vi "ti2_setYPos.vi"(8 "error in (no error)":errorcluster, 10 "speed":i32=4, 11 "y Position (um)":dbl) -> (0 "error out":errorcluster)   [LabVIEW 2018, in "ti2lv.lvlib"]
uses:
  ti2lv.lvlib
  ti2wrap/x64/Release/ti2wrap.dll
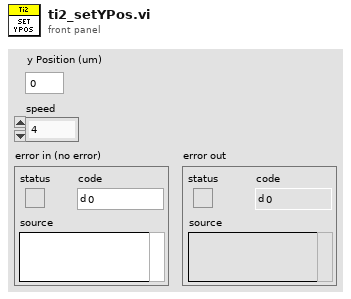
[diagram p1: front panel]
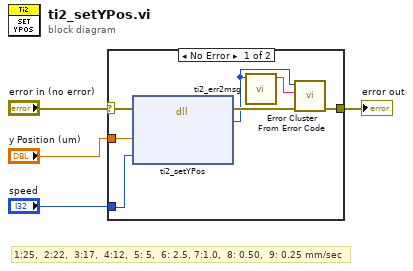
[diagram p0: block diagram]
diagram:
  # "1:25,  2:22, \t3:17,  4:12,\t\t5: 5,  6: 2.5,\t7:1.0,  8: 0.50,  9: 0.25 mm/sec"
  n1 = case shown="No Error" "error in (no error)" {
    selector: "error in (no error)" -> [w10 w12]
    tunnel: [w11 w12] -> w4
    tunnel: "y Position (um)" -> [w6 _]
    tunnel: "speed" -> [w5 _]
    frame No Error {
      n2 = dll-call lib="C:/LVCUR/Flash Gordon v0.6.1b/Hardware/Ti2/ti2wrap/x64/Release/ti2wrap.dll" fn="ti2_setYPos"(error in=w10, "yPos_um"=w6, "speed"=w5) -> (error out=w9:errorcluster, "return type"=w8:i32)  [unwired: 4 in, 1 out]
      n3 = call "ti2_err2msg.vi"("Error Code"=w8) -> ("Error Message"=w7:string)  [unwired: 10 in]
      n4 = call <vilib>:"Error Cluster From Error Code.vi"("error in (no error)"=w9, "error message (\"\")"=w7, "error code (0)"=w8) -> ("error out"=w11:errorcluster)  [unwired: 6 in]
    }
    frame Error {
    }
  }
  "error out" <- w4
